vi "lookupNodeReply.vi"(2 "node":string, 3 "Master":refnum<class "ROS_Master.lvclass">) -> (1 "XML":string)   [LabVIEW 2012, in "ROS_Master.lvclass"]
uses:
  <userlib>/ROSforLV/ROS/Code/ROS_Master/ROS_Master.lvclass
  <userlib>/ROSforLV/ROS/Code/ROS_Master/ROS_Master.lvclass/ROS_Master.ctl
panel:
  out "Master out":refnum<class "ROS_Master.lvclass">
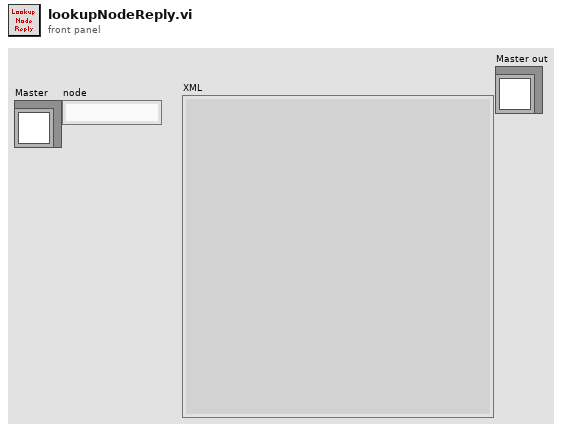
[diagram p1: front panel]
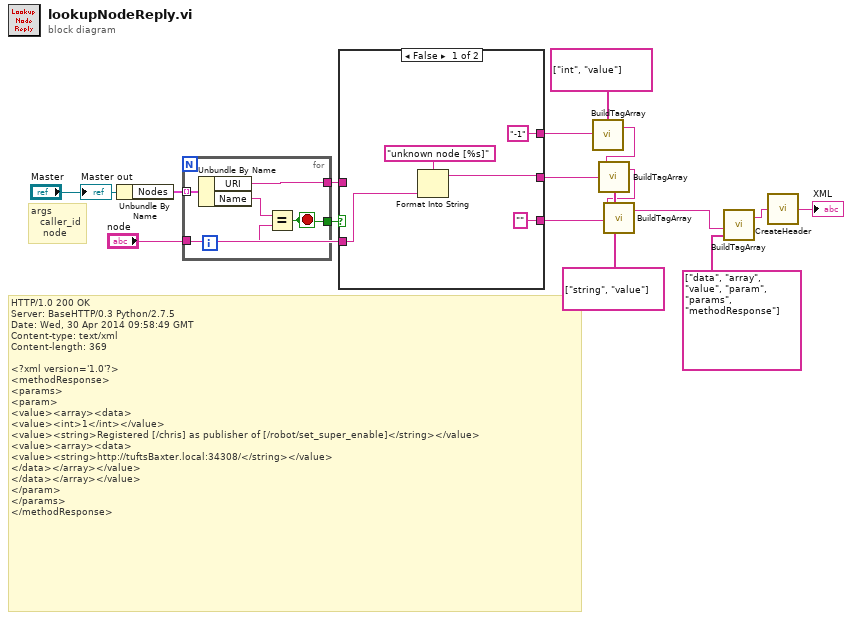
[diagram p0: block diagram]
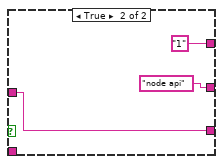
[diagram p2: hidden frame]
diagram:
  w6 = string[] ["string", "value"] ("tags")
  # "args\n   caller_id\n    node"
  # "HTTP/1.0 200 OK\nServer: BaseHTTP/0.3 Python/2.7.5\nDate: Wed, 30 Apr 2014 09:58:49 GMT\nContent-type: text/xml\nContent-length: 369\n\n<?xml version='1.0'?>\n<methodResponse>\n<params>\n<param>\n<value><array><data>\n<value><int>1</int></value>\n<value><string>Registered [/chris] as publisher of [/robot/set_super_enable]</string></value>\n<value><array><data>\n<value><string>http://tuftsBaxter.local:34308/</string></value>\n</data></array></value>\n</data></array></value>\n</param>\n</params>\n</methodResponse>"
  n1 = Unbundle By Name("Master") -> ("Nodes"=w11:cluster{"Name":string, "URI":string}[])
  n2 = for {
    tunnel: w11 -> [w21] mode=indexing
    tunnel: "node" -> [w19]
    tunnel: [w18] -> w10
    tunnel: [w17] -> w9
    stop <- w18 stop-if-true
    n3 = Unbundle By Name(w21) -> ("URI"=w17:string, "Name"=w20:string)
    n4 = Equal?(x=w20, y=w19) -> (x = y?=w18:bool)
  }
  n5 = case shown="False" w10 {
    tunnel: w9 -> [_ w28]
    tunnel: "node" -> [w24 _]
    tunnel: ["-1" ("value") "1" ("value")] -> w4
    tunnel: ["" ("URI") w28] -> w3
    tunnel: [w23 "node api" ("value")] -> w2
    frame False {
      n6 = Format Into String(format string="unknown node [%s]", w24) -> (resulting string=w23:string)  [unwired: 2 in, 1 out]
    }
    frame True {
    }
  }
  n7 = call <userlib>:"BuildTagArray.vi"("tags"=string[] ["int", "value"], "value"=w4) -> ("string out"=w15:string)  [unwired: 2 in]
  n8 = call <userlib>:"BuildTagArray.vi"("tags"=w6, "value"=w2, "string in"=w15) -> ("string out"=w5:string)  [unwired: 1 in]
  n9 = call <userlib>:"BuildTagArray.vi"("tags"=w6, "value"=w3, "string in"=w5) -> ("string out"=w1:string)  [unwired: 1 in]
  n10 = call <userlib>:"BuildTagArray.vi"("tags"=string[] ["data", "array", "value", "param", "params", "methodResponse"], "value"=w1) -> ("string out"=w13:string)  [unwired: 2 in]
  n11 = call <userlib>:"CreateHeader.vi"("Content"=w13) -> ("XML"=→"XML":string)
  "Master out" <- "Master"
